vi "Tree.vi"   [LabVIEW 2009, in "MicroDAQ.lvlib"]
uses:
  <instrlib>/MicroDAQ/MicroDAQ.lvlib
  <instrlib>/MicroDAQ/Channel/Analog Input/Read 1Chan 1Samp 1D SGL.vi
  <instrlib>/MicroDAQ/Channel/Analog Input/Analog Input.lvclass
  <instrlib>/MicroDAQ/Channel/Channel.lvclass
  <instrlib>/MicroDAQ/Channel/Analog Output/AO Configure Channel.vi
  <instrlib>/MicroDAQ/Channel/Analog Output/Analog output.lvclass
  <instrlib>/MicroDAQ/Channel/Analog Output/Write NChan NSamp 2D SGL.vi
  <instrlib>/MicroDAQ/Channel/Analog Input/Triggering External start.vi
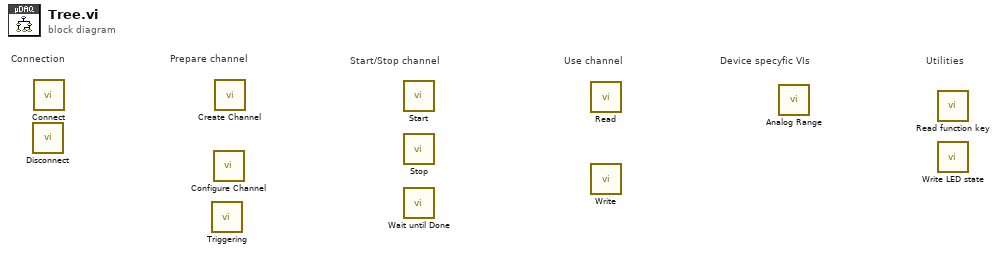
[diagram p0: block diagram]
diagram:
  # "Utilities"
  # "Device specyfic VIs"
  # "Start/Stop channel"
  # "Use channel"
  # "Prepare channel"
  # "Connection"
  n1 = call <instrlib>:"Disconnect.vi"() -> ()  [unwired: 11 in, 1 out]
  n2 = call <instrlib>:"Connect.vi"() -> ()  [unwired: 10 in, 2 out]
  n3 = call-poly <instrlib>:"Triggering.vi"() -> ()  [unwired: 10 in, 2 out]
  n4 = call-poly <instrlib>:"Configure Channel.vi"() -> ()  [unwired: 10 in, 2 out]
  n5 = call-poly <instrlib>:"Create Channel.vi"() -> ()  [unwired: 10 in, 2 out]
  n6 = call-dynamic "Start.vi"() -> ()  [unwired: 10 in, 2 out]
  n7 = call-dynamic "Stop.vi"() -> ()  [unwired: 10 in, 2 out]
  n8 = call-dynamic "Wait until Done.vi"() -> ()  [unwired: 10 in, 2 out]
  n9 = call-poly <instrlib>:"Read.vi"() -> ()  [unwired: 9 in, 3 out]
  n10 = call-poly <instrlib>:"Write.vi"() -> ()  [unwired: 10 in, 2 out]
  n11 = call <instrlib>:"Analog Range.vi"() -> ()  [unwired: 11 in, 1 out]
  n12 = call <instrlib>:"Read function key.vi"() -> ()  [unwired: 9 in, 3 out]
  n13 = call <instrlib>:"Write LED state.vi"() -> ()  [unwired: 10 in, 2 out]
